vi "DSF.Engine.Execution.Builder.Build.vi"(8 "error in (no error)":errorcluster, 9 "Transfer ID":i32, 10 "Plugin ID":i32, 11 "Builder in":refnum<class "DSF.Engine.Execution.Builder.lvclass">) -> (0 "error out":errorcluster, 3 "Builder out":refnum<class "DSF.Engine.Execution.Builder.lvclass">)   [LabVIEW 2016, in "DSF.Engine.lvlib" / "DSF.Engine.Execution.Builder.lvclass"]
uses:
  DSF.Engine.Execution.Builder.lvclass
  Cache/DSF.Engine.Memory.Cache.Framework.lvclass
  Cache/DSF.Engine.Memory.Cache.Plugin.lvclass
  Buffer/DSF.Engine.Memory.Buffer.lvclass
  Pointer/DSF.Engine.Memory.Pointer.VS Channels.lvclass
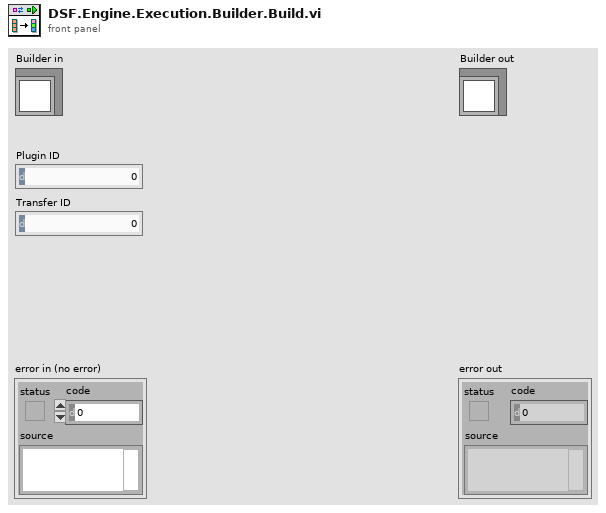
[diagram p1: front panel]
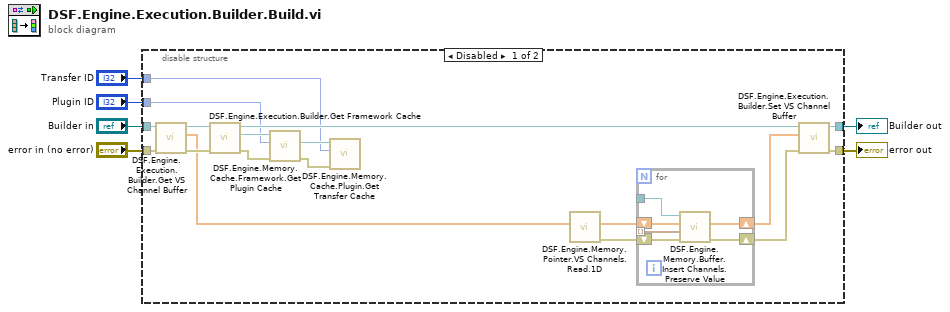
[diagram p0: block diagram]
diagram:
  n1 = disable-structure shown="Disabled" {
    disable-tunnel: [w29 w37] -> w6
    disable-tunnel: [w28 w36] -> w5
    disable-tunnel: "Builder in" -> [w27 w37]
    disable-tunnel: "error in (no error)" -> [w26 w36]
    disable-tunnel: "Plugin ID" -> [w9 _]
    disable-tunnel: "Transfer ID" -> [w8 _]
    frame Disabled {
      n2 = call "DSF.Engine.Execution.Builder.Get VS Channel Buffer.vi"("error in (no error)"=w26, "Builder in"=w27) -> ("error out"=w17:errorcluster, "VS Channel Buffer"=w16:dbl[], "Builder out"=w18:refnum<class "DSF.Engine.Execution.Builder.lvclass">)  [unwired: 7 in]
      n3 = call "DSF.Engine.Execution.Builder.Get Framework Cache.vi"("error in (no error)"=w17, "Builder in"=w18) -> ("error out"=w21:errorcluster, "Framework Cache"=w24:refnum<class "DSF.Engine.Memory.Cache.Framework.lvclass">, "Builder out"=w10:refnum<class "DSF.Engine.Execution.Builder.lvclass">)  [unwired: 7 in]
      n4 = call "DSF.Engine.Memory.Cache.Framework.Get Plugin Cache.vi"("error in (no error)"=w21, "Plugin ID"=w9, "Framework Cache in"=w24) -> ("error out"=w22:errorcluster, "Plugin Cache"=w23:refnum<class "DSF.Engine.Memory.Cache.Plugin.lvclass">)  [unwired: 6 in, 1 out]
      n5 = call "DSF.Engine.Memory.Cache.Plugin.Get Transfer Cache.vi"("error in (no error)"=w22, "Transfer ID"=w8, "Plugin Cache in"=w23) -> ("Transfer Cache"=w20:refnum<class "DSF.Engine.Memory.Cache.Transfer.lvclass">)  [unwired: 6 in, 2 out]
      n6 = call "DSF.Engine.Memory.Pointer.VS Channels.Read.1D.vi"("Channels Array in"=w16) -> ("error out"=w14:errorcluster, "Channels Array out"=w19:dbl[], "error in (no error)"=w25:errorcluster, "VS Channels Pointer in"=w12:refnum<class "DSF.Engine.Memory.Pointer.VS Channels.lvclass">)  [unwired: 5 in, 2 out]
      n7 = for {
        tunnel: [w30] -> w7 mode=indexing
        shift-right: [w33] -> w15
        shift-left: w19 -> [w34]
        shift-right: [w32] -> w13
        shift-left: w14 -> [w35]
        tunnel: [w31] -> w11
        n8 = call "DSF.Engine.Memory.Buffer.Insert Channels.Preserve Value.vi"("error in (no error)"=w35, "Channel Configuration"=w30, "VS Channels Array in"=w34, "Buffer in"=w31) -> ("error out"=w32:errorcluster, "VS Channels Array out"=w33:dbl[])  [unwired: 5 in, 1 out]
      }
      n9 = call "DSF.Engine.Execution.Builder.Set VS Channel Buffer.vi"("error in (no error)"=w13, "VS Channel Buffer"=w15, "Builder in"=w10) -> ("error out"=w28:errorcluster, "Builder out"=w29:refnum<class "DSF.Engine.Execution.Builder.lvclass">)  [unwired: 7 in]
    }
    frame Enabled {
    }
  }
  "error out" <- w5
  "Builder out" <- w6
